vi "File Manager.vi"(6 "File Functions":T4(ring), 8 "error in (no error)":errorcluster, 11 "array in":T1) -> (0 "error out":errorcluster, 1 "cancelled":bool, 3 "array out":T1)   [LabVIEW 2014]
uses:
  Libraries/Map Data Folder/All-Lines.ctl
  Libraries/Map Data Folder/LineCluster.ctl
  Libraries/Map Data Folder/LineConnection.ctl
  Libraries/Map Data Folder/Map Data.lvlib
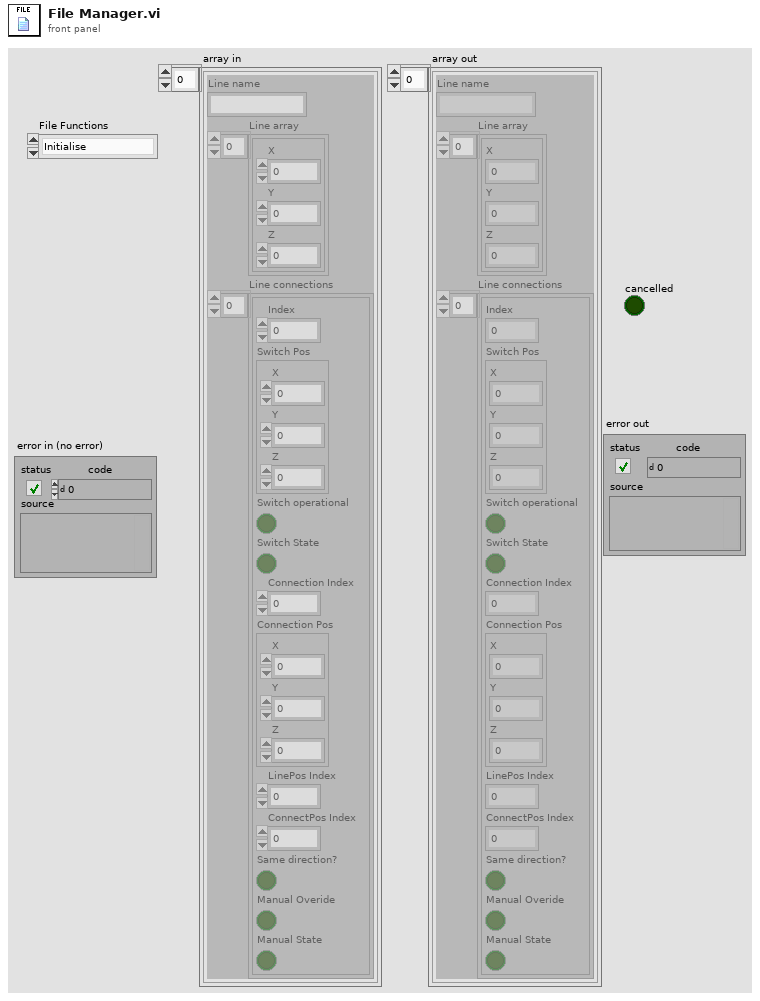
[diagram p1: front panel]
types:
  T1 = typedef "Map Data.lvlib/All-Lines.ctl" = T2[]
  T2 = typedef "Map Data.lvlib/LineCluster.ctl" = cluster{"Line name":string, "Line array":cluster{"X":dbl, "Y":dbl, "Z":dbl}[], "Line connections":T3[]}
  T3 = typedef "Map Data.lvlib/LineConnection.ctl" = cluster{"Index":i32, "Switch Pos":cluster{"X":dbl, "Y":dbl, "Z":dbl}, "Switch operational":bool, "Switch State":bool, "Connection Index":i32, "Connection Pos":cluster{"X":dbl, "Y":dbl, "Z":dbl}, "LinePos Index":i32, "ConnectPos Index":i32, "Same direction?":bool, "Manual Overide":bool, "Manual State":bool}
  T4 = enum16{"Initialise", "Close", "Read", "Write", "Ask for File", ""}
  T5 = enum16{"open", "replace", "create", "open or create", "replace or create", "replace or create with confirmation"}
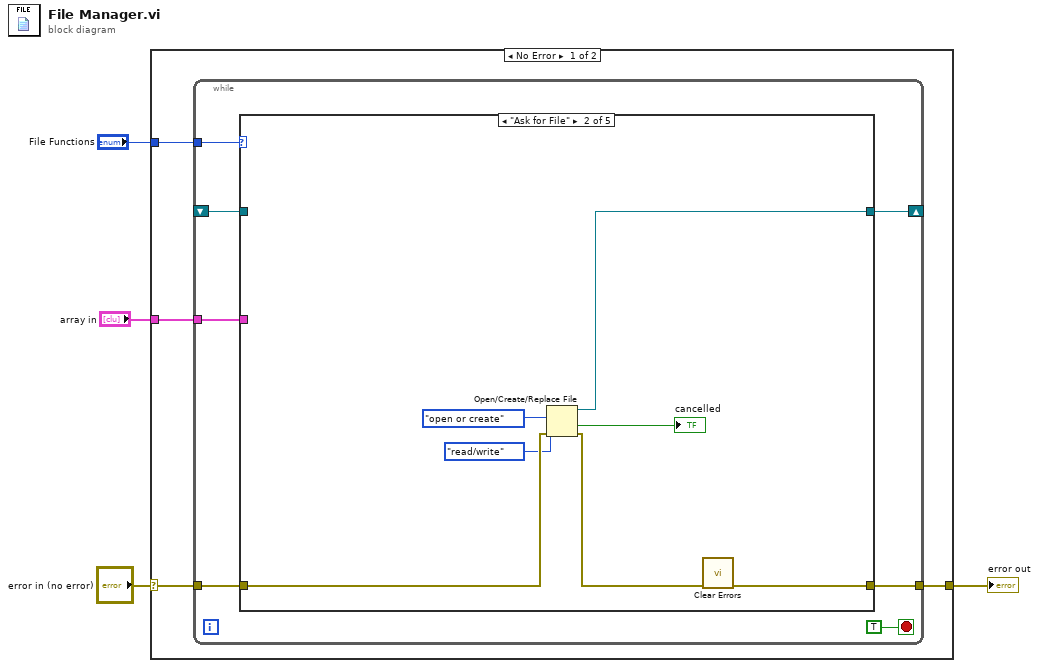
[diagram p0: block diagram]
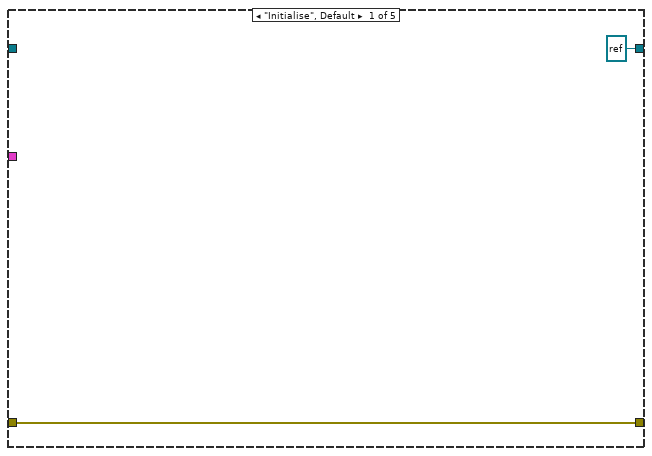
[diagram p2: hidden frame]
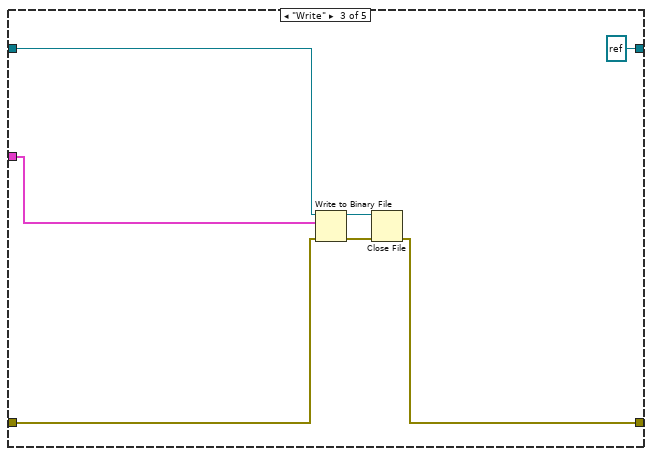
[diagram p3: hidden frame]
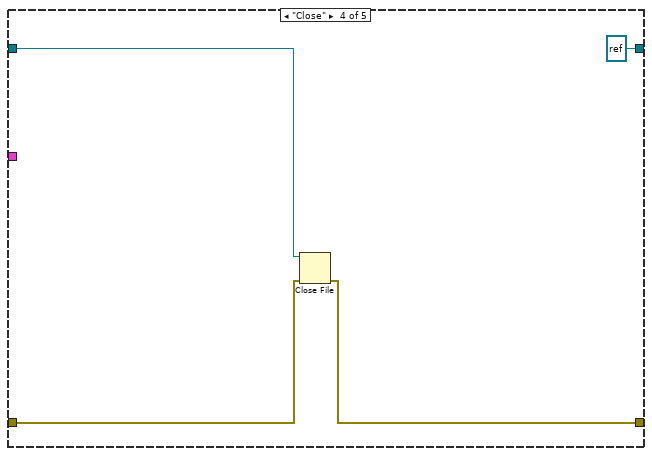
[diagram p4: hidden frame]
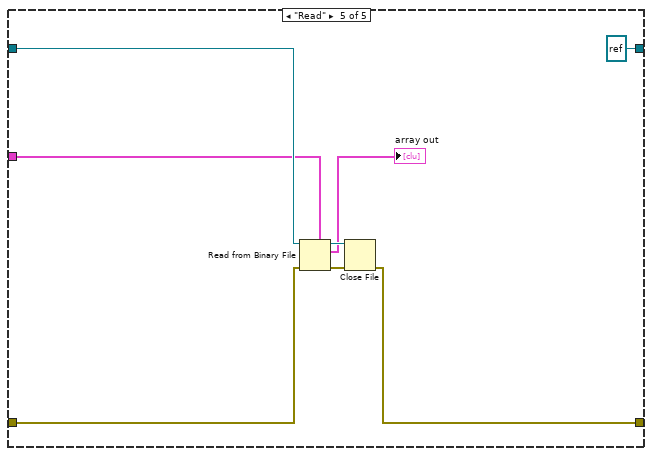
[diagram p5: hidden frame]
diagram:
  n1 = case shown="No Error" "error in (no error)" {
    selector: "error in (no error)" -> [w8 w44]
    tunnel: [w7 w44] -> w3
    tunnel: "File Functions" -> [w6 _]
    tunnel: "array in" -> [w5 _]
    frame No Error {
      n2 = while {
        tunnel: w8 -> [w14]
        tunnel: [w13] -> w7
        tunnel: w6 -> [w12]
        shift-right: [w11] -> _
        shift-left: _ -> [w10]
        tunnel: w5 -> [w9]
        stop <- TRUE stop-if-true
        n3 = case shown="\"Ask for File\"" w12 {
          tunnel: w14 -> [w17 w24 w30 w33 w43]
          tunnel: [w17 w18 w27 w32 w39] -> w13
          tunnel: [refnum<file> refnum ("refnum out") w20 refnum<file> refnum ("refnum out") refnum<file> refnum ("refnum out") refnum<file> refnum ("refnum out")] -> w11
          tunnel: w10 -> [_ _ w31 w35 w41]
          tunnel: w9 -> [_ _ w25 _ w37]
          frame "Initialise", Default {
          }
          frame "Ask for File" {
            n4 = Open/Create/Replace File(error in=w24, operation (0:open)=T5."open or create", access (0:read/write)=enum16{"read/write", "read-only", "write-only"}."read/write") -> (refnum out=w20:refnum<file>, cancelled=→"cancelled":bool, error out=w23:errorcluster)  [unwired: 3 in]
            n5 = call <vilib>:"Clear Errors.vi"("error in (no error)"=w23) -> ("error out"=w18:errorcluster)  [unwired: 5 in, 1 out]
          }
          frame "Write" {
            n6 = Write to Binary File(file (use dialog)=w31, data=w25, error in=w30) -> (refnum out=w28:refnum<file>, error out=w29:errorcluster)  [unwired: 3 in, 1 out]
            n7 = Close File(refnum=w28, error in=w29) -> (error out=w27:errorcluster)  [unwired: 1 out]
          }
          frame "Close" {
            n8 = Close File(refnum=w35, error in=w33) -> (error out=w32:errorcluster)  [unwired: 1 out]
          }
          frame "Read" {
            n9 = Read from Binary File(5:w37, 8:w43, 11:w41) -> (0:w40:errorcluster, 2:→"array out":T1, 3:w42:refnum<file>)  [unwired: 3 in, 1 out]
            n10 = Close File(refnum=w42, error in=w40) -> (error out=w39:errorcluster)  [unwired: 1 out]
          }
        }
      }
    }
    frame Error {
    }
  }
  "error out" <- w3
